vi "Set Visible.vi"(8 "error in (no error)":errorcluster, 10 "Show? [T]":bool=TRUE, 11 "MMI Scaling in":refnum<class "IContainer.lvclass">) -> (0 "error out":errorcluster, 3 "MMI Scaling out":refnum<class "IContainer.lvclass">)   [LabVIEW 2013, in "IContainer.lvclass"]
doc: "Copyright 2018, Wiebe Walstra, wiebe@carya.nl."
uses:
  IContainer.lvclass
  IObject.lvclass
  IContainer.lvclass/IContainer.ctl
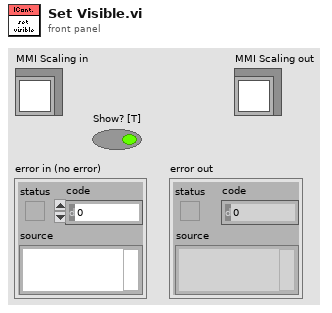
[diagram p1: front panel]
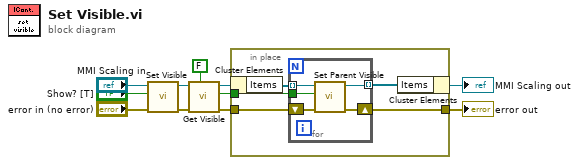
[diagram p0: block diagram]
diagram:
  n1 = call-parent "Set Visible.vi"("error in (no error)"="error in (no error)", "Show? [T]"="Show? [T]", "MMI Scaling in"="MMI Scaling in") -> ("error out"=w5:errorcluster, "MMI Scaling out"=w4:refnum<class "IContainer.lvclass">)  [unwired: 7 in]
  n2 = call-dynamic "Get Visible.vi"("Hide if children are hidden? [T]"=FALSE, "error in (no error)"=w5, "IContainer in"=w4) -> ("error out"=w8:errorcluster, "Visible?"=w6:bool, "IContainer out"=w7:refnum<class "IContainer.lvclass">)  [unwired: 5 in, 1 out]
  n3 = in-place {
    in-place-border: [w16] -> w2
    in-place-border: w8 -> [w15]
    in-place-border: w6 -> [w12]
    n4 = in-place-cluster #1(w7) -> ("Items"=w14:refnum<class "IObject.lvclass">[])
    n5 = for {
      tunnel: [w18] -> w13 mode=indexing
      tunnel: w14 -> [w20] mode=indexing
      shift-right: [w17] -> w16
      shift-left: w15 -> [w21]
      tunnel: w12 -> [w19]
      n6 = call-dynamic "Set Parent Visible.vi"("error in (no error)"=w21, "Parent visible? [T]"=w19, "IObject in"=w20) -> ("error out"=w17:errorcluster, "IObject out"=w18:refnum<class "IObject.lvclass">)  [unwired: 7 in]
    }
    n7 = in-place-cluster #1("Items"=w13) -> (→"MMI Scaling out":refnum<class "IContainer.lvclass">)
  }
  "error out" <- w2
